vi "Destroy BufferMap.vi"(8 "error in":errorcluster, 9 "Return Elements (T)":bool=TRUE, 11 "Buffer":refnum<data-value>) -> (0 "error out":errorcluster, 2 "buffers":refnum<data-value>[](array[refnum]), 3 "Names":string[](array[string]))   [LabVIEW 2013, in "CircularBuffer.lvlib" / "VariantBufferMap.lvclass"]
doc: "This VI releases resources that have been created for the ring buffer."
uses:
  VariantBufferMap.lvclass
  VariantBuffer/VariantBuffer.lvclass
  VariantBufferMap.lvclass/VariantBufferMap.ctl
  VariantBuffer/WriteBufferError.vi
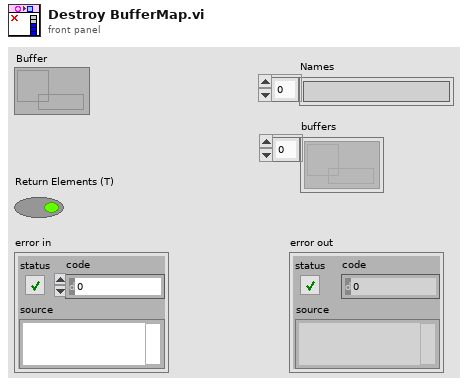
[diagram p1: front panel]
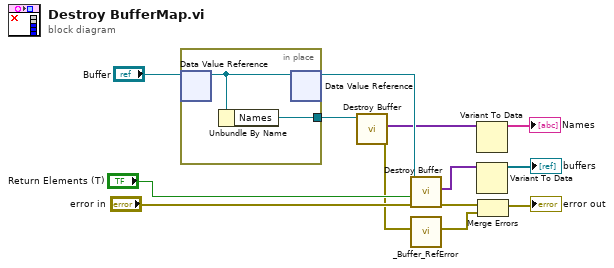
[diagram p0: block diagram]
diagram:
  n1 = in-place {
    in-place-border: [w15] -> w13
    n2 = in-place-dvr #1("Buffer") -> (w14:refnum<class "VariantBufferMap.lvclass">)  [unwired: 1 out]
    n3 = Unbundle By Name(w14) -> ("Names"=w15:refnum<data-value>)
    n4 = in-place-dvr #1(w14) -> (w8:refnum<data-value>)  [unwired: 1 out]
  }
  n5 = call "Destroy Buffer.vi"("Buffer"=w13) -> ("error out"=w6:errorcluster, "elements"=w2:variant[])  [unwired: 9 in]
  n6 = call "Destroy Buffer.vi"("error in"="error in", "Return Elements (T)"="Return Elements (T)", "Buffer"=w8) -> ("error out"=w4:errorcluster, "elements"=w11:variant[])  [unwired: 7 in]
  n7 = call "_Buffer_RefError.vi"("error in (no error)"=w6) -> ("error out"=w5:errorcluster)  [unwired: 10 in]
  n8 = Variant To Data(Variant=w2) -> (data=→"Names":string[])  [unwired: 2 in, 1 out]
  n9 = Variant To Data(Variant=w11) -> (data=→"buffers":refnum<data-value>[])  [unwired: 2 in, 1 out]
  n10 = Merge Errors(w4, w5) -> (→"error out":errorcluster)
